vi "completed chain.vi"(9 "longueur":i32, 10 "Combler par":u8=32, 11 "Chaine":string="A1B2C3D4E5F6G7H8I9J1K2L3M") -> (3 "chaîne":string)   [LabVIEW 2020, in "Library Commun.lvlib"]
uses:
  Library Commun.lvlib
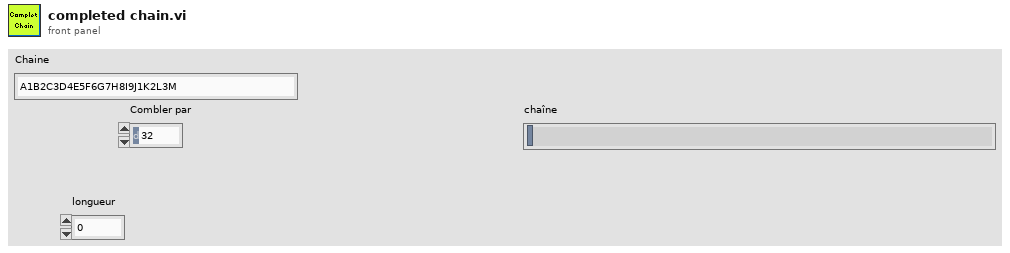
[diagram p1: front panel]
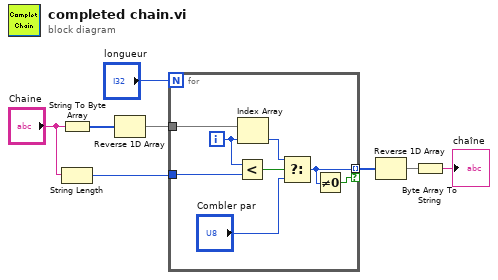
[diagram p0: block diagram]
diagram:
  n1 = String To Byte Array(string="Chaine") -> (unsigned byte array=w6:u8[])
  n2 = String Length(string="Chaine") -> (length=w5:i32)
  n3 = Reverse 1D Array(array=w6) -> (reversed array=w2:u8[])
  n4 = for {
    N: "longueur" -> [_]
    tunnel: w2 -> [w16]
    tunnel: w5 -> [w14]
    tunnel: [w10] -> w4 mode=indexing if=w9
    i -> [w15]
    n5 = Less?(x=w15, y=w14) -> (x < y?=w13:bool)
    n6 = Index Array(array=w16, index=w15) -> (element=w12:u8)
    n7 = Select(t=w12, s=w13, f="Combler par") -> (s? t:f=w10:u8)
    n8 = Not Equal To 0?(x=w10) -> (x != 0?=w9:bool)
  }
  n9 = Reverse 1D Array(array=w4) -> (reversed array=w1:u8[])
  n10 = Byte Array To String(unsigned byte array=w1) -> (string=→"chaîne":string)
